vi "PS_LCR_cal.vi"(10 "Lower Voltge Limit":dbl=1.2, 11 "Upper Voltage Limit":dbl=4.0) -> (0 "Min":dbl, 1 "XY Graph":cluster{"Y":dbl[], "Y":dbl[]}[](graph)=[{"Y"=[0.0, 0.05, 0.1, 0.15, 0.2, 0.25, 0.3, 0.35, 0.4, 0.45, 0.5, 0.55, 0.6, 0.65, 0.7, 0.75, 0.8, 0.85, 0.9, 0.95, 1.0, 1.05, 1.1, 1.15, 1.2, 1.25, 1.3, 1.35, 1.4, 1.45, 1.5, 1.55, 1.6, 1.65, 1.7, 1.75, 1.8, 1.85, 1.9, 1.95, 2.0, 2.05, 2.1, 2.15, 2.2, 2.25, 2.3, 2.35, 2.4, 2.45, 2.5, 2.55, 2.6, 2.65, 2.7, 2.75, 2.8, 2.85, 2.9, 2.95, 3.0, 3.05, 3.1, 3.15, 3.2, 3.25, 3.3, 3.35, 3.4, 3.45, 3.5, 3.55, 3.6, 3.65, 3.7, 3.75, 3.8, 3.85, 3.9, 3.95, 4.0, 4.05, 4.1, 4.15, 4.2, 4.25, 4.3, 4.35, 4.4, 4.45, 4.5, 4.55, 4.6, 4.65, 4.7, 4.75, 4.8, 4.85, 4.9, 4.95, 5.0, 5.05], "Y"=[1.5298757135269085, 1.5328388976296985, 1.5293925856704482, 1.5345781578612852, 1.5339661959375244, 1.53018169447358, 1.5265743399104366, 1.5220007296691076, 1.51427068423586, 1.5063957004884947, 1.4997124321084379, 1.4819977450237825, 1.4447163815532993, 1.3573024588883174, 1.161603516393886, 0.820918029268634, 0.4199061821541399, 0.153622585843183, 0.15030511317271325, 0.43882866711630325, 0.9999006895515649, 1.7411958476019447, 2.5304981523045864, 3.255995414422078, 3.818694517751893, 4.165918458818913, 4.28151481082073, 4.198819455810404, 3.959059256056534, 3.6098544367966032, 3.1979556371752222, 2.7795023464614927, 2.353174058815591, 1.9588288800544416, 1.6140365864269837, 1.3070571708940657, 1.0370854125367381, 0.8146051627749571, 0.6324661084613775, 0.488896759796258, 0.3677123343585585, 0.27295498563700904, 0.2089245346149273, 0.1557966576810819, 0.11780676597356136, 0.09493875253211967, 0.08471256374939808, 0.07883451829497443, 0.07988129347656164, 0.08679000994821919, 0.1060506744395145, 0.11840262266212312, 0.14189870211324745, 0.16217393518736928, 0.18887475937212259, 0.21549506349261563, 0.24541673756696256, 0.27099026846865953, 0.29912437444837736, 0.32951307523590956, 0.3613189505652336, 0.3922229898377022, 0.4230787177962361, 0.44779873039006196, 0.4836145678075603, 0.509687339034607, 0.5342946249192798, 0.5705774896484697, 0.6011594528745015, 0.6259599926645998, 0.6571217110122272, 0.6779283991150254, 0.7090740151905816, 0.7342932688254709, 0.7632809176513753, 0.787839898681874, 0.815201020034375, 0.8366357778752933, 0.8612269695320995, 0.891003730987698, 0.9074461724203882, 0.9323916595874564, 0.957933004817351, 0.981493527508089, 1.0035080424099714, 1.0244435728298853, 1.046007169575612, 1.0641888732873335, 1.082000179455684, 1.1046749711119777, 1.124096703595656, 1.14831750481961, 1.1598159438564613, 1.180815894520082, 1.2004630880208707, 1.2108342296260255, 1.2341531943794966, 1.245104089613326, 1.2719659918665696, 1.2829813044791825, 1.3021775805287772, 1.3143201915840468]}], 2 "Min Voltage":dbl, 3 "Max Voltage":dbl)   [LabVIEW 2011]
uses:
  PS_Global.vi
  <vilib>/Instr/_visa.llb/VISA Configure Serial Port (Instr).vi
  <vilib>/Analysis/NI_AALBase.lvlib
panel:
  in  "Stop at Voltage":dbl=4.0
  in  "Number of Points":dbl=100.0
  out "Max":dbl
  out "Waveform Chart 2":dbl(graph)
  in  "baud rate":u32=115200
  out "Waveform Chart":dbl(graph)
  out "Signal Mean":dbl format="%0.2f"
  out "Voltage 2 Setpoint":dbl
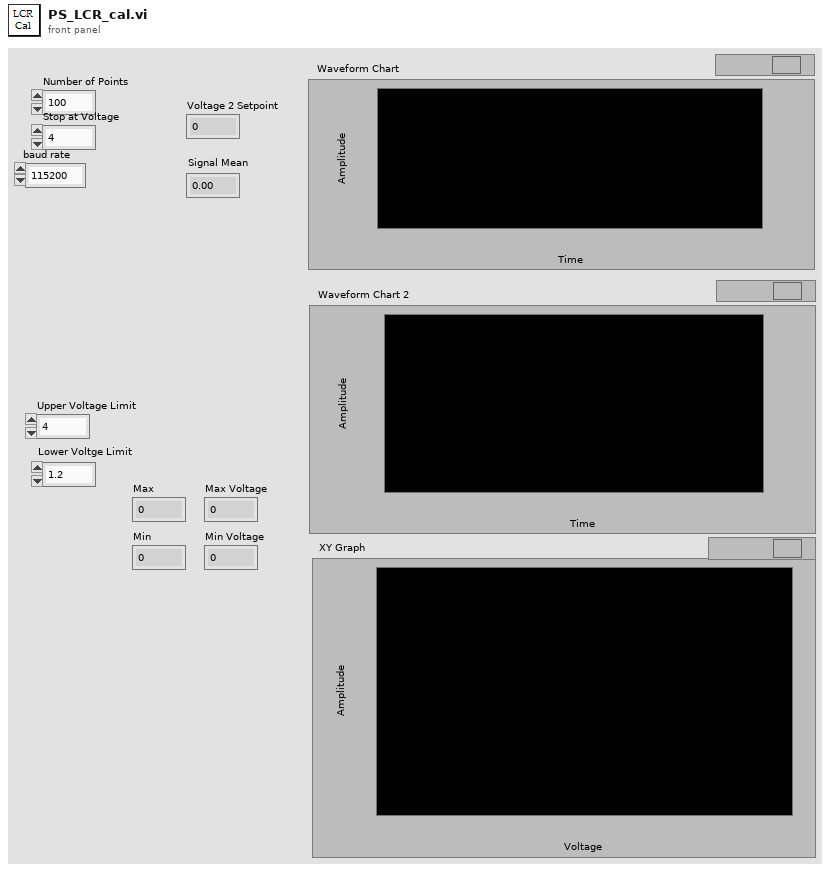
[diagram p1: front panel]
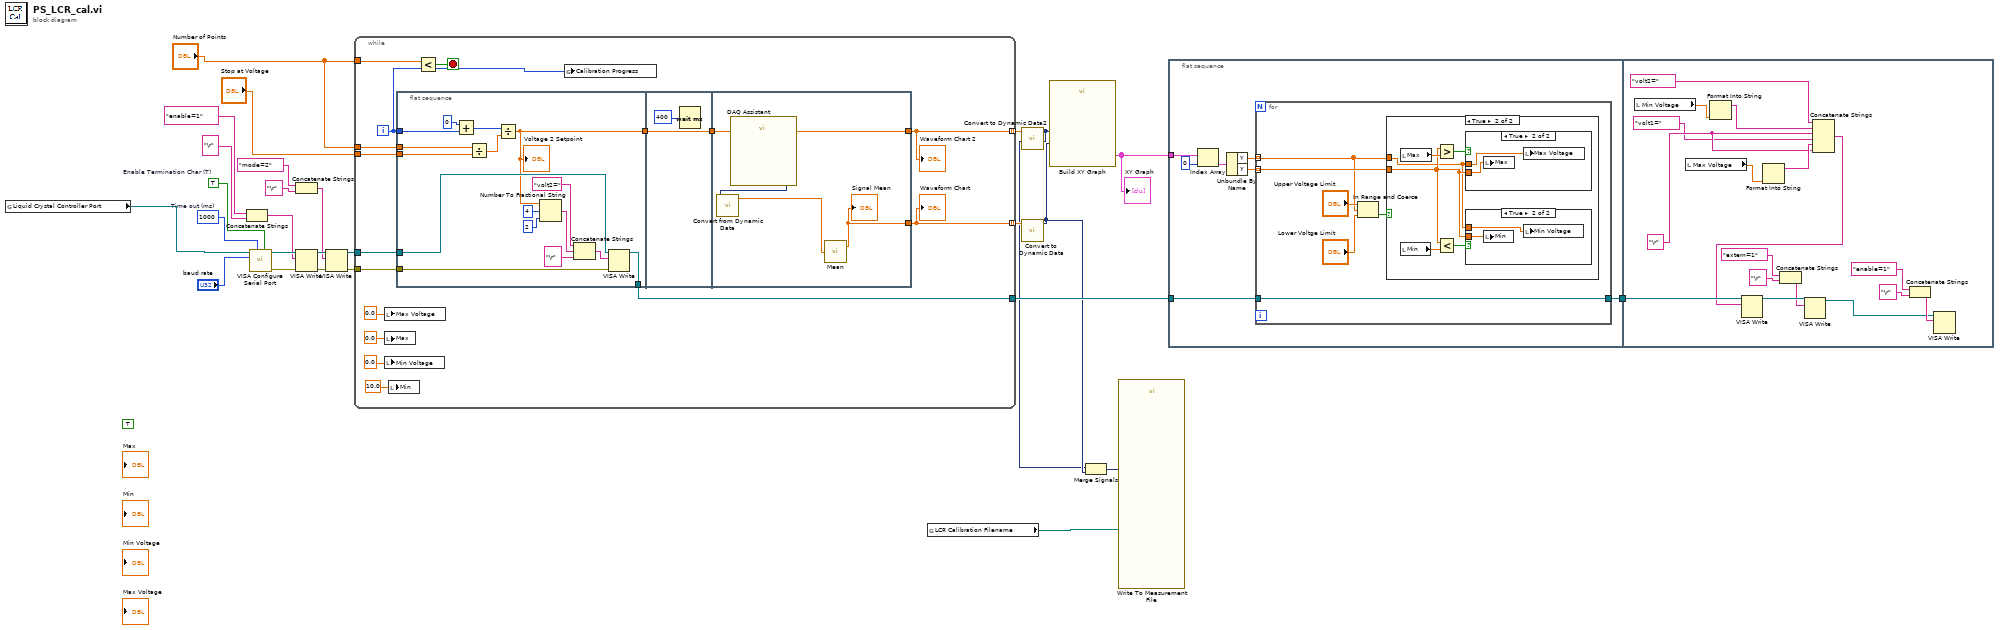
[diagram p0: block diagram]
diagram:
  (unwired) TRUE
  w23 = TRUE  # Enable Termination Char (T)
  w26 = 1000  # Time out (ms)
  n1 = global read "PS_Global.vi" "Liquid Crystal Controller Port"() -> (w4:refnum<visa-resource-name>)
  n2 = Concatenate Strings("enable=1", "\r") -> (w20:string)
  n3 = call-poly "VISA Configure Serial Port"("VISA resource name"=w4, "timeout (10sec)"=w26, "Enable Termination\nChar (T)"=w23, "baud rate (9600)"="baud rate") -> ("VISA resource name out"=w25:refnum<visa-resource-name>, "error out"=w24:errorcluster)  [unwired: 10 in]
  n4 = Concatenate Strings("mode=2" ("write buffer"), "\r") -> (w16:string)
  n5 = VISA Write(VISA resource name=w25, write buffer=w20, error in (no error)=w24) -> (VISA resource name out=w17:refnum<visa-resource-name>, error out=w15:errorcluster)  [unwired: 1 out]
  n6 = VISA Write(VISA resource name=w17, write buffer=w16, error in (no error)=w15) -> (VISA resource name out=w13:refnum<visa-resource-name>, error out=w14:errorcluster)  [unwired: 1 out]
  n7 = while {
    tunnel: w13 -> [w42]
    tunnel: w14 -> [w41]
    tunnel: [w38] -> w12 mode=indexing
    tunnel: [w37] -> w11 mode=indexing
    tunnel: [w32] -> w9
    tunnel: "Number of Points" -> [w30]
    tunnel: "Number of Points" -> [w29]
    tunnel: "Stop at Voltage" -> [w28]
    i -> [w31]
    stop <- w43 stop-if-true
    n8 = local write "Max Voltage"(0.0 ("Max Voltage")) -> ()
    n9 = local write "Max"(0.0 ("Max")) -> ()
    n10 = local write "Min Voltage"(0.0 ("Min Voltage")) -> ()
    n11 = local write "Min"(10.0 ("Min")) -> ()
    n12 = flat-sequence {
      tunnel: w31 -> [w51]
      tunnel: w42 -> [w57]
      tunnel: w41 -> [w56]
      tunnel: [w48] -> w39
      tunnel: [w47] -> w32
      tunnel: w29 -> [w45]
      tunnel: w28 -> [w44]
      tunnel: [w60] -> w40
      tunnel: w39 -> [w60]
      tunnel: w40 -> [w63]
      tunnel: [w64] -> w38
      tunnel: [w63] -> w37
      frame #0 {
        n13 = Add(x=0, y=w51) -> (x+y=w52:i32)
        n14 = Divide(x=w45, y=w44) -> (x/y=w46:dbl)
        n15 = Divide(x=w52, y=w46) -> (x/y=w48:dbl)
        "Voltage 2 Setpoint" <- w48
        n16 = Number To Fractional String(number=w48, width (-)=i16 4, precision (6)=i16 2) -> (F-format string=w55:string)  [unwired: 1 in]
        n17 = Concatenate Strings("volt2=" ("string"), w55, "\r") -> (w58:string)
        n18 = VISA Write(VISA resource name=w57, write buffer=w58, error in (no error)=w56) -> (VISA resource name out=w47:refnum<visa-resource-name>)  [unwired: 2 out]
      }
      frame #1 {
        n19 = Wait (ms)(milliseconds to wait=u32 400) -> ()  [unwired: 1 out]
      }
      frame #2 {
        n20 = call "DAQ Assistant"() -> ("data"=w65:dynamicdata)  [unwired: 17 in, 2 out]
        n21 = call "Convert from Dynamic Data"("Dynamic Data Type"=w65) -> ("Array"=w62:dbl[])  [unwired: 3 in]
        n22 = call <vilib>:"Mean.vi"("X"=w62) -> ("mean"=w64:dbl)  [unwired: 1 out]
        "Signal Mean" <- w64
      }
    }
    n23 = Less?(x=w30, y=w31) -> (x < y?=w43:bool)
    n24 = global write "PS_Global.vi" "Calibration Progress"(w31) -> ()
    "Waveform Chart" <- w38
    "Waveform Chart 2" <- w37
  }
  n25 = global read "PS_Global.vi" "LCR Calibration Filename"() -> (w1:path)
  n26 = call "Convert to Dynamic Data2"("Array"=w11) -> ("Dynamic Data Type"=w6:dynamicdata)  [unwired: 3 in]
  n27 = call "Convert to Dynamic Data"("Array"=w12) -> ("Dynamic Data Type"=w7:dynamicdata)  [unwired: 3 in]
  n28 = call "Build XY Graph"("Y Input"=w7, "X Input"=w6) -> ("XY Graph"=w10:cluster{"Y":dbl[], "Y":dbl[]}[])  [unwired: 3 in, 6 out]
  "XY Graph" <- w10
  n29 = Merge Signals(w6, w7) -> (w5:dynamicdata)
  n30 = call "Write To Measurement File"("Signals"=w5, "Filename"=w1) -> ()  [unwired: 15 in, 3 out]
  n31 = flat-sequence {
    tunnel: w10 -> [w72]
    tunnel: w9 -> [w67]
    tunnel: [w66] -> w8
    tunnel: w8 -> [w105]
    frame #0 {
      n32 = Index Array(array=w72, index=0) -> (element=w70:cluster{"Y":dbl[], "Y":dbl[]})
      n33 = Unbundle By Name(w70) -> ("Y"=w69:dbl[], "Y"=w68:dbl[])
      n34 = for {
        tunnel: w69 -> [w74] mode=indexing
        tunnel: w68 -> [w75] mode=indexing
        tunnel: w67 -> [w73]
        tunnel: [w73] -> w66
        n35 = In Range and Coerce(upper limit="Upper Voltage Limit", x=w74, lower limit="Lower Voltge Limit") -> (In Range?=w78:bool)  [unwired: 1 out]
        n36 = case shown="True" w78 {
          tunnel: w75 -> [_ w80]
          tunnel: w74 -> [_ w79]
          frame False {
          }
          frame True {
            n37 = local read "Max"() -> (w82:dbl)
            n38 = local read "Min"() -> (w83:dbl)
            n39 = Greater?(x=w80, y=w82) -> (0:w81:bool)
            n40 = Less?(x=w80, y=w83) -> (x < y?=w84:bool)
            n41 = case shown="True" w81 {
              tunnel: w80 -> [_ w88]
              tunnel: w79 -> [_ w87]
              frame False {
              }
              frame True {
                n42 = local write "Max"(w88) -> ()
                n43 = local write "Max Voltage"(w87) -> ()
              }
            }
            n44 = case shown="True" w84 {
              tunnel: w80 -> [_ w86]
              tunnel: w79 -> [_ w85]
              frame False {
              }
              frame True {
                n45 = local write "Min"(w86) -> ()
                n46 = local write "Min Voltage"(w85) -> ()
              }
            }
          }
        }
      }
    }
    frame #1 {
      w98 = "\r"
      n47 = local read "Min Voltage"() -> (w103:dbl)
      n48 = local read "Max Voltage"() -> (w100:dbl)
      n49 = Format Into String(w103) -> (resulting string=w101:string)  [unwired: 3 in, 1 out]
      n50 = Format Into String(w100) -> (resulting string=w99:string)  [unwired: 3 in, 1 out]
      n51 = Concatenate Strings("extern=1" ("write buffer"), "\r") -> (w93:string)
      n52 = Concatenate Strings("volt2=" ("write buffer"), w101, w98, "volt1=" ("write buffer"), w99, w98) -> (w104:string)
      n53 = VISA Write(VISA resource name=w105, write buffer=w104) -> (VISA resource name out=w96:refnum<visa-resource-name>)  [unwired: 1 in, 2 out]
      n54 = VISA Write(VISA resource name=w96, write buffer=w93) -> (VISA resource name out=w89:refnum<visa-resource-name>)  [unwired: 1 in, 2 out]
      n55 = Concatenate Strings("enable=1" ("write buffer"), "\r") -> (w92:string)
      n56 = VISA Write(VISA resource name=w89, write buffer=w92) -> ()  [unwired: 1 in, 3 out]
    }
  }
